vi "Fast Remove Item Property FuncGlobal.vi"(5 "Action":enum16{"Open or Add", "Close Ref"}(ring), 8 "error in (no error)":errorcluster, 10 "Property Name":string, 11 "Item Ref in":T1 format="%.0x") -> (0 "error out":errorcluster, 1 "Removed":bool, 3 "Item Ref out":T1 format="%.0x")   [LabVIEW 2011]
doc: "Removes the <B>Property Name</B> from an item."
uses:
  <vilib>/NI Veristand/Custom Device API/Custom Device Item Ref.ctl
  <vilib>/NI Veristand/Custom Device API/Custom Device API.lvlib
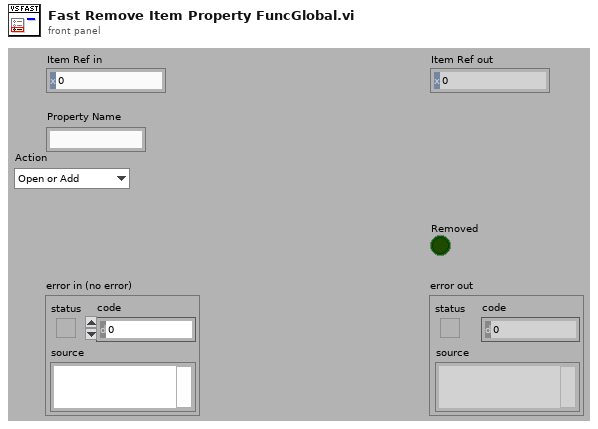
[diagram p1: front panel]
types:
  T1 = typedef "Custom Device API.lvlib/Custom Device Item Ref.ctl" = u64
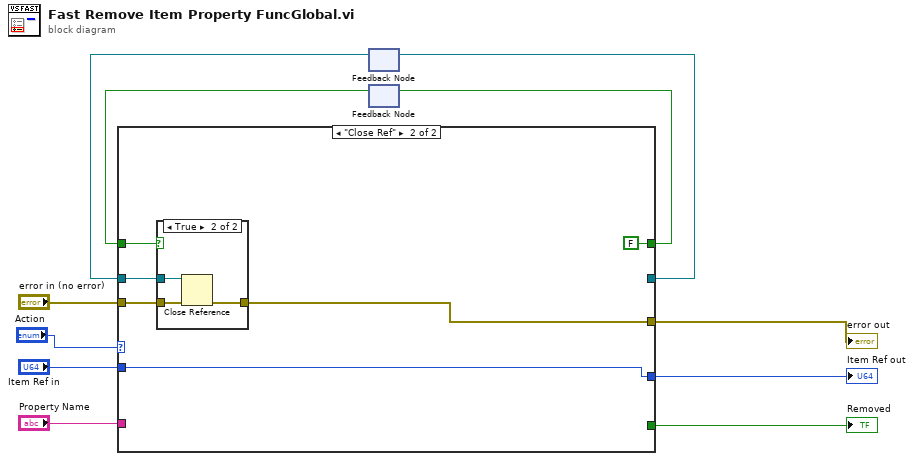
[diagram p0: block diagram]
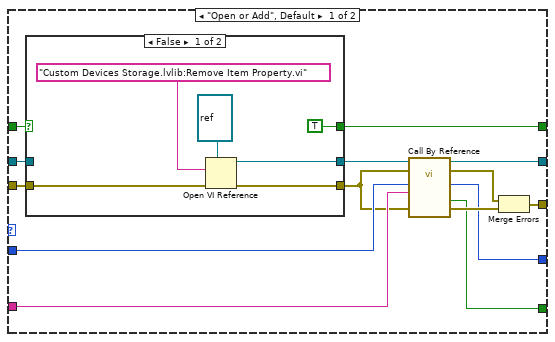
[diagram p2: hidden frame]
diagram:
  n1 = feedback #1() -> (w2:refnum<vi>)  [unwired: 1 in]
  n2 = feedback #2() -> (w3:bool)  [unwired: 1 in]
  n3 = case shown="\"Close Ref\"" "Action" {
    tunnel: [w24 _] -> w5
    tunnel: [w23 w37] -> w11
    tunnel: "Item Ref in" -> [w22 w35]
    tunnel: "Property Name" -> [w21 _]
    tunnel: [w20 w35] -> w8
    tunnel: [w19 _] -> w7
    tunnel: "error in (no error)" -> [w18 w39]
    tunnel: [w14 FALSE] -> w4
    tunnel: w3 -> [w13 w38]
    tunnel: w2 -> [w12 w40]
    frame "Open or Add", Default {
      n4 = case shown="False" w13 {
        selector: w13 -> [_ w34]
        tunnel: w18 -> [w29 w32]
        tunnel: [w28 w32] -> w17
        tunnel: [w27 w33] -> w16
        tunnel: [TRUE w34] -> w14
        tunnel: w12 -> [_ w33]
        frame False {
          n5 = Open VI Reference(type specifier VI Refnum (for type only)=refnum<vi> refnum, vi path="Custom Devices Storage.lvlib:Remove Item Property.vi", error in (no error)=w29) -> (vi reference=w27:refnum<vi>, error out=w28:errorcluster)  [unwired: 3 out]
        }
        frame True {
        }
      }
      n6 = call-by-ref "?"(reference=w16, error in=w17, 8:"error in (no error)"=w17, "Property Name"=w21, "Item Ref in"=w22) -> (reference out=w24:refnum<vi>, error out=w15:errorcluster, 0:"error out"=w25:errorcluster, "Removed"=w19:bool, "Item Ref out"=w20:T1)  [unwired: 6 in]
      n7 = Merge Errors(w15, w25) -> (w23:errorcluster)
    }
    frame "Close Ref" {
      n8 = case shown="True" w38 {
        tunnel: w40 -> [_ w44]
        tunnel: w39 -> [w41 w43]
        tunnel: [w41 w42] -> w37
        frame False {
        }
        frame True {
          n9 = Close Reference(reference=w44, error in (no error)=w43) -> (error out=w42:errorcluster)
        }
      }
    }
  }
  "Item Ref out" <- w8
  "error out" <- w11
  "Removed" <- w7
  n10 = feedback-in #1(w5) -> ()
  n11 = feedback-in #2(w4) -> ()
